vi "Go to Idle.vi"(8 "error in (no error)":errorcluster, 11 "Idle in":refnum<class "Idle.lvclass">) -> (0 "error out":errorcluster, 3 "State Actor.lvclass":refnum<class "State Actor.lvclass">)   [LabVIEW 2024, in "Test States.lvlib" / "Idle.lvclass"]
uses:
  Idle.lvclass
  C:/Program Files/National Instruments/LabVIEW 2024/vi.lib/ni/Actors/State Actor/State Actor/State Actor.lvclass
  <vilib>/ni/Actors/State Actor/State Actor/State Actor.lvclass
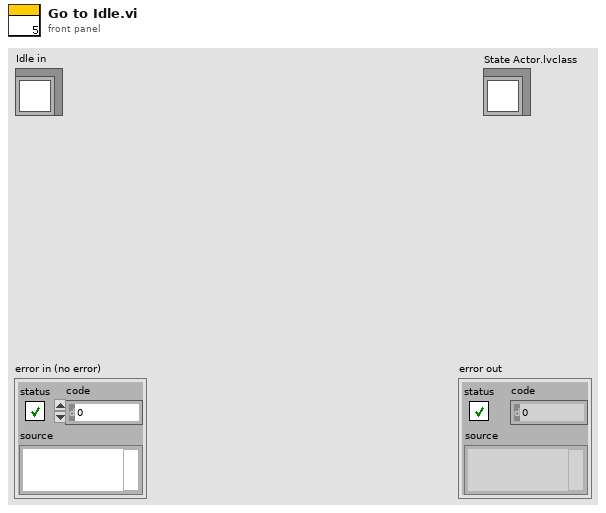
[diagram p1: front panel]
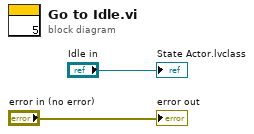
[diagram p0: block diagram]
diagram:
  "error out" <- "error in (no error)"
  "State Actor.lvclass" <- "Idle in"
